vi "Certificate(RGT).vi"(2 "select":enum16{"Setup", "Add-on", "Search", "Release"}(ring), 5 "key":string, 11 "error in":errorcluster) -> (4 "Certificate":u8, 6 "found":bool, 15 "error out":errorcluster)   [LabVIEW 2011]
uses:
  <vilib>/Utility/NIReport.llb/NI_report.lvclass
  <vilib>/addons/_office/excel.llb/Excel Get Data (str).vi
  <vilib>/addons/_office/excel.llb/Excel Find and Replace (str).vi
  <vilib>/addons/_office/NI_ReportGenerationToolkit.lvlib
  <vilib>/Utility/NIReport.llb/Excel/NI_Excel.lvclass
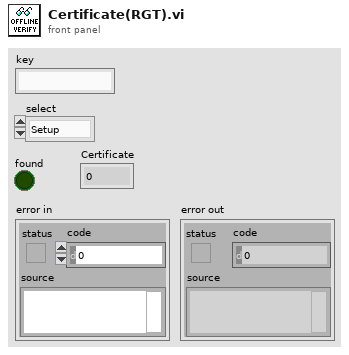
[diagram p1: front panel]
types:
  T1 = enum16{"maximized", "minimized", "normal", "no change"}
  T2 = enum16{"Standard Report", "HTML", "Word", "Excel"}
  T3 = cluster{"position (Excel)":cluster{"row":i32, "column":i32}, "name (Excel)":string, "bookmark (Word)":string}
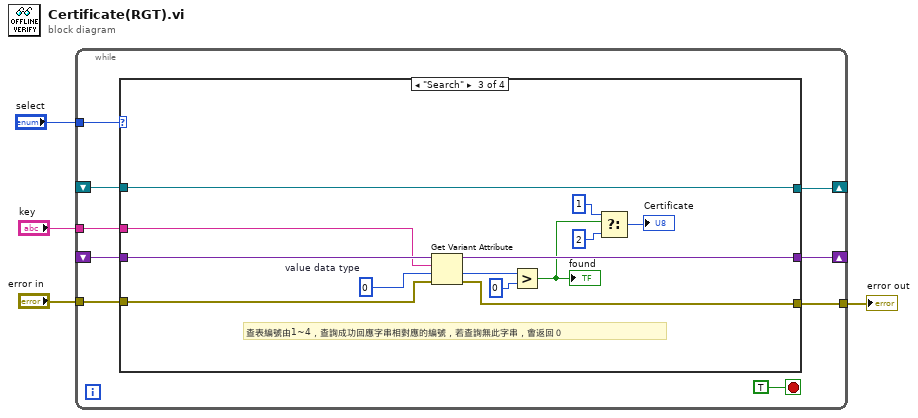
[diagram p0: block diagram]
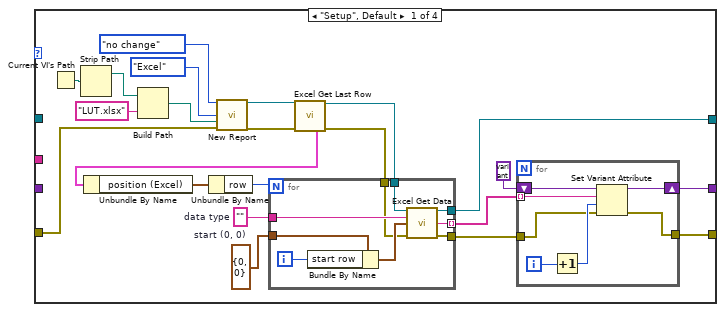
[diagram p2: hidden frame]
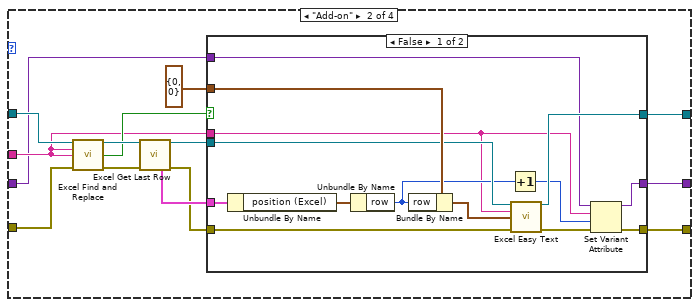
[diagram p3: hidden frame]
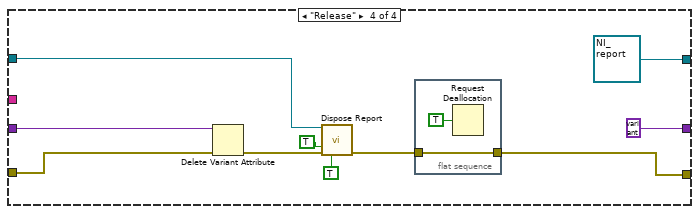
[diagram p5: hidden frame]
diagram:
  n1 = while {
    shift-right: [w13] -> _
    shift-left: _ -> [w12]
    shift-right: [w10] -> _
    shift-left: _ -> [w9]
    tunnel: "key" -> [w8]
    tunnel: "select" -> [w7]
    tunnel: [w6] -> w1
    tunnel: "error in" -> [w5]
    stop <- TRUE stop-if-true
    n2 = case shown="\"Search\"" w7 {
      tunnel: [w34 w52 w93 variant ("variant")] -> w13
      tunnel: w12 -> [_ w53 w94 w105]
      tunnel: [w18 w54 w87 refnum<class "NI_report.lvclass"> refnum ("report out")] -> w10
      tunnel: w9 -> [_ w65 w87 w100]
      tunnel: w8 -> [_ w57 w90 _]
      tunnel: [w14 w55 w88 w97] -> w6
      tunnel: w5 -> [w17 w56 w89 w103]
      frame "Setup", Default {
        w33 = ""  # data type
        w32 = cluster{"start row":i32, "start column":i32} {"start row"=0, "start column"=0}  # start (0, 0)
        n3 = Current VI's Path() -> (path=w28:path)
        n4 = Strip Path(path=w28) -> (stripped path=w27:path)  [unwired: 1 out]
        n5 = Build Path(base path=w27, name or relative path="LUT.xlsx") -> (appended path=w25:path)
        n6 = call <vilib>:"New Report.vi"("window state (normal)"=T1."no change", "report type"=T2."Excel", "template (empty)"=w25, "error in (no error)"=w17) -> ("report out"=w24:refnum<class "NI_report.lvclass">, "error out"=w23:errorcluster)  [unwired: 10 in]
        n7 = call <vilib>:"Excel Get Last Row.vi"("report in"=w24, "error in (no error)"=w23) -> ("report out"=w19:refnum<class "NI_report.lvclass">, "MS Office parameters out"=w20:T3, "error out"=w16:errorcluster)  [unwired: 11 in]
        n8 = Unbundle By Name(w20) -> ("position (Excel)"=w22:cluster{"row":i32, "column":i32})
        n9 = Unbundle By Name(w22) -> ("row"=w21:i32)
        n10 = for {
          N: w21 -> [_]
          tunnel: [w44] -> w31 mode=indexing
          tunnel: w33 -> [w43]
          tunnel: w32 -> [w42]
          tunnel: w19 -> [w39]
          tunnel: [w38] -> w18
          tunnel: w16 -> [w37]
          tunnel: [w36] -> w15
          i -> [w40]
          n11 = Bundle By Name(cluster=w42, "start row"=w40) -> (w41:cluster{"start row":i32, "start column":i32})
          n12 = call-poly <vilib>:"Excel Get Data.vi"("report in"=w39, "data type"=w43, "start (0, 0)"=w41, "error in (no error)"=w37) -> ("report out"=w38:refnum<class "NI_report.lvclass">, "data"=w44:string, "error out"=w36:errorcluster)  [unwired: 9 in]
        }
        n13 = for {
          shift-right: [w50] -> w34
          shift-left: variant ("variant") -> [w51]
          tunnel: w31 -> [w49] mode=indexing
          tunnel: w15 -> [w46]
          tunnel: [w45] -> w14
          i -> [w47]
          n14 = Increment(x=w47) -> (x+1=w48:i32)
          n15 = Set Variant Attribute(Variant=w51, name=w49, value=w48, error in=w46) -> (Variant out=w50:variant, error out=w45:errorcluster)  [unwired: 1 out]
        }
      }
      frame "Add-on" {
        n16 = call-poly <vilib>:"Excel Find and Replace.vi"("report in"=w65, "searched string"=w57, "replacement"=w57, "error in (no error)"=w56) -> ("report out"=w64:refnum<class "NI_report.lvclass">, "found?"=w63:bool, "error out"=w62:errorcluster)  [unwired: 9 in]
        n17 = call <vilib>:"Excel Get Last Row.vi"("report in"=w64, "error in (no error)"=w62) -> ("report out"=w58:refnum<class "NI_report.lvclass">, "MS Office parameters out"=w61:T3, "error out"=w60:errorcluster)  [unwired: 11 in]
        n18 = case shown="False" w63 {
          tunnel: w61 -> [w78 _]
          tunnel: w60 -> [w74 w82]
          tunnel: cluster{"row":i32, "column":i32} {"row"=0, "column"=0} ("start") -> [w77 _]
          tunnel: w58 -> [w75 w81]
          tunnel: w57 -> [w66 _]
          tunnel: [w68 w82] -> w55
          tunnel: [w73 w81] -> w54
          tunnel: w53 -> [w70 w80]
          tunnel: [w67 w80] -> w52
          frame False {
            n19 = Unbundle By Name(w78) -> ("position (Excel)"=w79:cluster{"row":i32, "column":i32})
            n20 = Unbundle By Name(w79) -> ("row"=w71:i32)
            n21 = Bundle By Name(cluster=w77, "row"=w71) -> (w76:cluster{"row":i32, "column":i32})
            n22 = Increment(x=w71) -> (x+1=w72:i32)
            n23 = call <vilib>:"Excel Easy Text.vi"("report in"=w75, "text"=w66, "start (-1, -1)"=w76, "error in (no error)"=w74) -> ("report out"=w73:refnum<class "NI_report.lvclass">, "error out"=w69:errorcluster)  [unwired: 7 in, 3 out]
            n24 = Set Variant Attribute(Variant=w70, name=w66, value=w72, error in=w69) -> (Variant out=w67:variant, error out=w68:errorcluster)  [unwired: 1 out]
          }
          frame True {
          }
        }
      }
      frame "Search" {
        w95 = 0  # value data type
        # "查表編號由1~4，查詢成功回應字串相對應的編號，若查詢無此字串，會返回０"
        n25 = Get Variant Attribute(Variant=w94, name=w90, default value (empty Variant)=w95, error in=w89) -> (duplicate Variant=w93:variant, value=w92:i32, error out=w88:errorcluster)  [unwired: 1 out]
        n26 = Greater?(x=w92, y=0) -> (0:w86:bool)
        "found" <- w86
        n27 = Select(t=u8 1, s=w86, f=u8 2) -> (s? t:f=→"Certificate":u8)
      }
      frame "Release" {
        n28 = Delete Variant Attribute(4:w103, 7:w105) -> (0:w101:errorcluster)  [unwired: 1 in, 2 out]
        n29 = call-dynamic "Dispose Report.vi"("report in"=w100, "save changes? (F)"=TRUE, "error in (no error)"=w101, "close report? (T)"=TRUE) -> ("error out"=w98:errorcluster)  [unwired: 11 in]
        n30 = flat-sequence {
          tunnel: w98 -> [w107]
          tunnel: [w107] -> w97
          frame #0 {
            n31 = Request Deallocation(TRUE ("flag")) -> ()
          }
        }
      }
    }
  }
  "error out" <- w1
